vi "Read (Multiple Digital Waveforms).vi"(0 "VISA resource name":refnum<visa-resource-name>, 1 "Segment Index (0)":i32 format="%.0g", 5 "Channels":i32[](array[ring])=[41, 42] items=["POD 1"=41, "POD 2"=42], 9 "Maximum Time (10000ms)":u32=10000, 11 "error in (no error)":errorcluster) -> (4 "VISA resource name out":refnum<visa-resource-name>, 6 "Digital Waveform Graph":digitalwaveform[](graph), 15 "error out":errorcluster)   [LabVIEW 2013, in "Agilent 90000 Series.lvlib"]
doc: "Initiates an acquisition on all channels that you enabled with the <B>Configure Channel</B> VI. The VI waits for the acquisition to complete and returns the waveform for the Source channel you specified. If the oscilloscope did not complete the acquisition within the time period you specify with the Timeout parameter, the VI returns a time out error. A common cause for a timeout error is the acquisition was not triggered. For example, the trigger level is out of range of the waveform.If the sampling mode is set to segment, you can set the <B>Segment Index</B>.\n\nCall the <B>Fetch (Digital Waveform)</B> VI to obtain the waveforms for each of the remaining enabled Source channels without initiating another acquisition.\n\nNote: If your instrument does not support auto compensation for probe attenuation, you may need to adjust the scaling of the Waveform Data accordingly. This is handled automatically in the <B>Configure Channel</B> VI or can be done manually by multiplying the Waveform Data by the probe attenuation."
uses:
  Agilent 90000 Series.lvlib
  Low Level/Fetch (Digital Waveform).vi
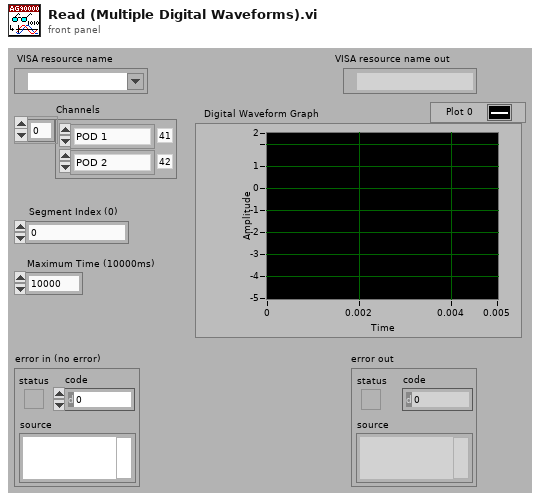
[diagram p1: front panel]
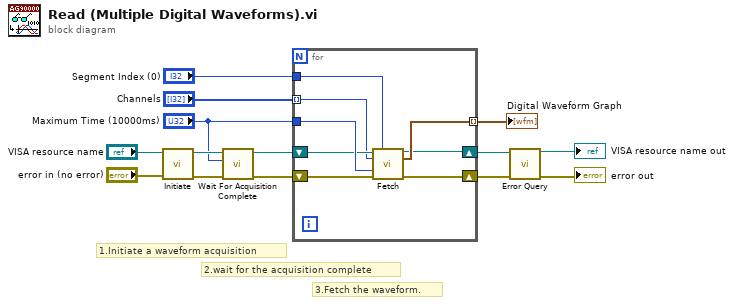
[diagram p0: block diagram]
diagram:
  # "3.Fetch the waveform."
  # "2.wait for the acquisition complete"
  # "1.Initiate a waveform acquisition"
  n1 = call "Initiate.vi"("error in (no error)"="error in (no error)", "VISA resource name"="VISA resource name") -> ("error out"=w7:errorcluster, "VISA resource name out"=w8:refnum<visa-resource-name>)  [unwired: 8 out]
  n2 = call "Wait For Acquisition Complete.vi"("error in (no error)"=w7, "Maximum Time (10000ms)"="Maximum Time (10000ms)", "VISA resource name"=w8) -> ("error out"=w5:errorcluster, "VISA resource name out"=w6:refnum<visa-resource-name>)  [unwired: 7 out]
  n3 = for {
    tunnel: "Segment Index (0)" -> [w16]
    tunnel: "Channels" -> [w15] mode=indexing
    shift-right: [w20] -> w10
    shift-left: w6 -> [w18]
    shift-right: [w19] -> w9
    shift-left: w5 -> [w17]
    tunnel: "Maximum Time (10000ms)" -> [w22]
    tunnel: [w21] -> w1 mode=indexing
    n4 = call-poly "Fetch.vi"("VISA resource name"=w18, "Segment Index (0)"=w16, "Channel (41: POD 1)"=w15, "Maximum Time (10000ms)"=w22, "error in (no error)"=w17) -> ("VISA resource name out"=w20:refnum<visa-resource-name>, "Digital Waveform Graph"=w21:digitalwaveform, "error out"=w19:errorcluster)  [unwired: 8 out]
  }
  "Digital Waveform Graph" <- w1
  n5 = call "Error Query.vi"("error in (no error)"=w9, "VISA resource name"=w10) -> ("error out"=→"error out":errorcluster, "VISA resource name out"=→"VISA resource name out":refnum<visa-resource-name>)  [unwired: 8 out]
